vi "XL320_Toggle Torque.vi"(8 "error in (no error)":errorcluster, 9 "Toggle torque (OFF)":bool, 10 "Motor ID (0)":u8, 11 "VISA resource name":refnum<visa-resource-name>) -> (0 "error out":errorcluster, 3 "VISA resource name out":refnum<visa-resource-name>)   [LabVIEW 2017, in "Dynamixel XL320.lvlib"]
doc: "Turns the motor's torque on or off."
uses:
  <instrlib>/Dynamixel XL320 (Drivers instrument)/Dynamixel XL320.lvlib
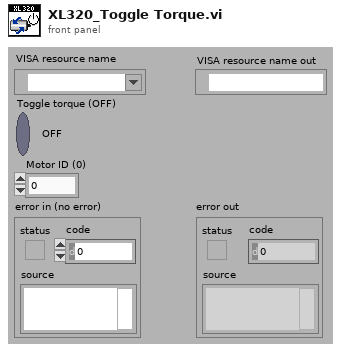
[diagram p1: front panel]
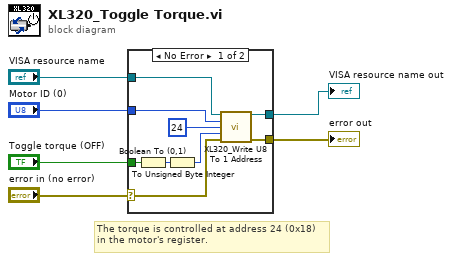
[diagram p0: block diagram]
diagram:
  # "The torque is controlled at address 24 (0x18)\nin the motor's register."
  n1 = case shown="No Error" "error in (no error)" {
    selector: "error in (no error)" -> [w12 w16]
    tunnel: "Toggle torque (OFF)" -> [w15 _]
    tunnel: "VISA resource name" -> [w14 w17]
    tunnel: [w11 w17] -> w4
    tunnel: [w10 w16] -> w3
    tunnel: "Motor ID (0)" -> [w13 _]
    frame No Error {
      n2 = Boolean To (0,1)(Boolean=w15) -> (0, 1=w8:i16)
      n3 = To Unsigned Byte Integer(number=w8) -> (unsigned 8bit integer=w7:u8)
      n4 = call <instrlib>:"XL320_Write U8 To 1 Address.vi"("VISA resource name"=w14, "Motor ID (0)"=w13, "Address number (0)"=u16 24, "Parameter (0)"=w7, "error in (no error)"=w12) -> ("VISA resource name out"=w11:refnum<visa-resource-name>, "error out"=w10:errorcluster)  [unwired: 9 in]
    }
    frame Error {
    }
  }
  "VISA resource name out" <- w4
  "error out" <- w3
